vi "Sauvegarde.vi"(11 "Table Control":string[][](array[string])) -> ()   [LabVIEW 2026]
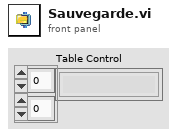
[diagram p1: front panel]
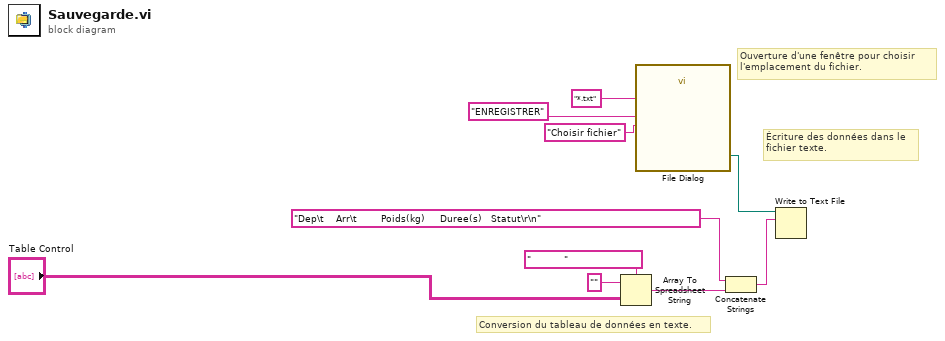
[diagram p0: block diagram]
diagram:
  # "Écriture des données dans le \nfichier texte."
  # "Ouverture d'une fenêtre pour choisir \nl'emplacement du fichier."
  # "Conversion du tableau de données en texte."
  n1 = Array To Spreadsheet String(delimiter (Tab)="           ", array="Table Control", 3:"" ("format string")) -> (spreadsheet string=w8:string)
  n2 = call "File Dialog"("prompt"="Choisir fichier", "button label"="ENREGISTRER", "pattern (all files)"="*.txt") -> ("selected path"=w4:path)  [unwired: 9 in, 3 out]
  n3 = Concatenate Strings("Dep\t    Arr\t        Poids(kg)     Duree(s)   Statut\r\n" ("string"), w8) -> (w9:string)
  n4 = Write to Text File(file (use dialog)=w4, text=w9) -> ()  [unwired: 2 in, 3 out]
